vi "Practicingeventhandler.vi"() -> ()   [LabVIEW 2020]
panel:
  in  "Boolean":bool
  in  "stop":bool
  out "x*y":dbl
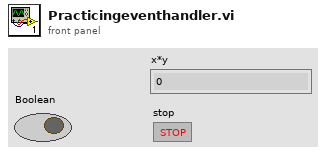
[diagram p1: front panel]
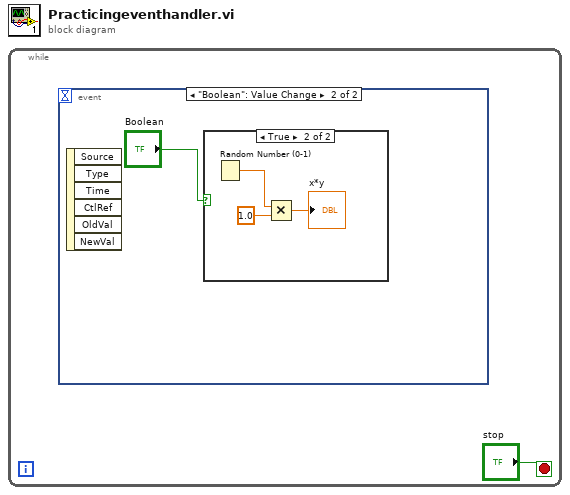
[diagram p0: block diagram]
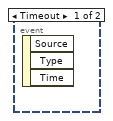
[diagram p2: hidden frame]
diagram:
  n1 = while {
    stop <- "stop" stop-if-true
    n2 = event shown="[1] \"Boolean\": Value Change" {
      selector: _ -> [_ _]
      dyn-events: _ -> [_ _]
      timeout: _ -> [_ _]
      event Timeout {
        n3 = event-data() -> ()  [unwired: 1 in, 3 out]
      }
      event "Boolean": Value Change {
        n4 = event-data() -> ()  [unwired: 1 in, 6 out]
        n5 = case shown="True" "Boolean" {
          frame False {
          }
          frame True {
            n6 = Random Number (0-1)() -> (number: 0 to 1=w4:dbl)
            n7 = Multiply(x=w4, y=1.0) -> (x*y=→"x*y":dbl)
          }
        }
      }
    }
  }
